vi "Write Top Level Value.vi"(7 "Key":string, 8 "error in (no error)":errorcluster, 10 "Value":variant, 11 "file path (use dialog)":path) -> (0 "error out":errorcluster)   [LabVIEW 2017, in "TOML.lvlib"]
uses:
  TOML.lvlib
  TOML Key-Value Pair.ctl
  TOML Value.ctl
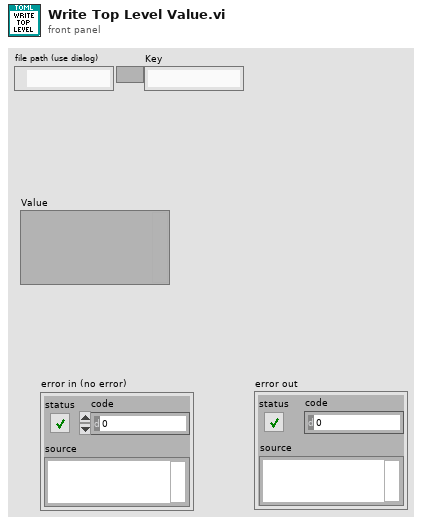
[diagram p1: front panel]
types:
  T1 = typedef "TOML.lvlib/TOML Key-Value Pair.ctl" = cluster{"Key":string, "Value":T2}
  T2 = typedef "TOML.lvlib/TOML Value.ctl" = cluster{"type":enum16{"Table", "Array", "String", "Integer", "Float", "Boolean", "Offset Date-Time", "Local Date-Time", "Local Date", "Local Time"}, "value":variant}
  T3 = enum16{"open", "replace", "create", "open or create", "replace or create", "replace or create with confirmation"}
  T4 = enum16{"Table", "Array", "String", "Integer", "Float", "Boolean", "Offset Date-Time", "Local Date-Time", "Local Date", "Local Time"}
  T5 = cluster{"type":enum16{"Table", "Array", "String", "Integer", "Float", "Boolean", "Offset Date-Time", "Local Date-Time", "Local Date", "Local Time"}, T1[]}
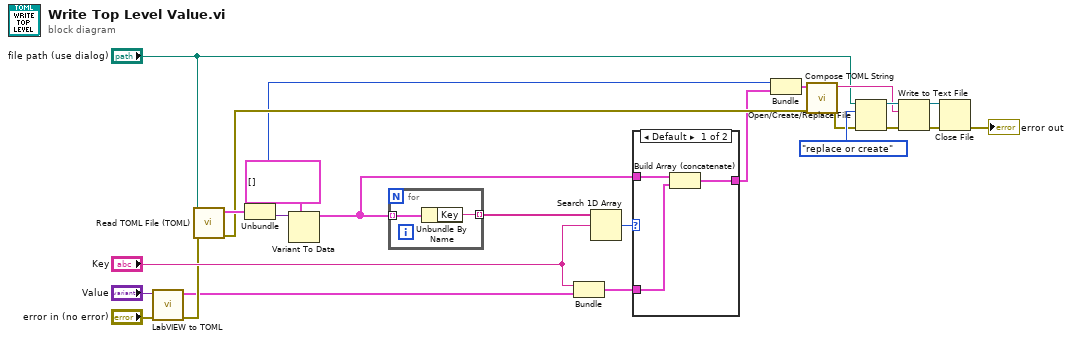
[diagram p0: block diagram]
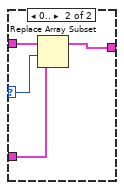
[diagram p2: hidden frame]
diagram:
  n1 = call "LabVIEW to TOML.vi"("error in (no error)"="error in (no error)", "LV Value"="Value") -> ("error out"=w8:errorcluster, "TOML Value"=w6:T2)  [unwired: 8 in]
  n2 = call "Read TOML File (TOML).vi"("error in (no error)"=w8, "file path (use dialog)"="file path (use dialog)") -> ("error out"=w7:errorcluster, "Value"=w14:T2)  [unwired: 8 in]
  n3 = Unbundle(w14) -> ("type"=w3:T4, "value"=w13:variant)
  n4 = Variant To Data(type=T1[] [], Variant=w13) -> (data=w4:T1[])  [unwired: 1 in, 1 out]
  n5 = for {
    tunnel: w4 -> [w27] mode=indexing
    tunnel: [w26] -> w11 mode=indexing
    n6 = Unbundle By Name(w27) -> ("Key"=w26:string)
  }
  n7 = Bundle("Key"="Key", "TOML Value"=w6) -> (w5:cluster{"Key":string, "TOML Value":T2})  [unwired: 1 in]
  n8 = Search 1D Array(1D array=w11, element="Key") -> (index of element=w10:i32)  [unwired: 1 in]
  n9 = case shown="Default" w10 {
    selector: w10 -> [_ w33]
    tunnel: w4 -> [w30 w34]
    tunnel: [w29 w32] -> w2
    tunnel: w5 -> [w28 w31]
    frame Default {
      n10 = Build Array (concatenate)(w30, w28) -> (w29:T1[])
    }
    frame 0.. {
      n11 = Replace Array Subset(array=w34, new element=w31, index=w33) -> (w32:T1[])
    }
  }
  n12 = Bundle("type"=w3, w2) -> (w1:T5)  [unwired: 1 in]
  n13 = call "Compose TOML String.vi"("error in (no error)"=w7, "Value"=w1) -> ("error out"=w17:errorcluster, "String"=w18:string)  [unwired: 8 in]
  n14 = Open/Create/Replace File(file path (use dialog)="file path (use dialog)", error in=w17, operation (0:open)=T3."replace or create") -> (refnum out=w23:refnum<file>, error out=w24:errorcluster)  [unwired: 3 in, 1 out]
  n15 = Write to Text File(file (use dialog)=w23, text=w18, error in=w24) -> (refnum out=w21:refnum<file>, error out=w22:errorcluster)  [unwired: 1 in, 1 out]
  n16 = Close File(refnum=w21, error in=w22) -> (error out=→"error out":errorcluster)  [unwired: 1 out]
